vi "StartClone.vi"(7 "ShowPanel?":bool, 8 "error in (no error)":errorcluster, 10 "ModuleName":string="unnamed", 11 "VI Refnum":refnum<vi>) -> (0 "error out":errorcluster, 1 "FlagImpairBroadcast":T1, 3 "ModuleAdmin":refnum<class "ModuleAdmin.lvclass">)   [LabVIEW 2017, in "FlagImpairModule.lvlib"]
uses:
  FlagImpairModule.lvlib
  Protected/Broadcasts/clBroadcastEvents.ctl
  Protected/clEventType.ctl
  <userlib>/NIST/ModuleAdminLib/ModuleAdmin/ModuleAdmin.lvclass
  C:/Program Files (x86)/National Instruments/LabVIEW 2017/user.lib/NIST/ModuleAdminLib/ModuleAdminBase/ModuleAdminBase.lvclass
  <userlib>/NIST/ModuleAdminLib/CloneRegistration/CloneRegistration.lvclass
  <userlib>/NIST/ModuleAdminLib/ModuleAdmin/ModuleAdmin.lvclass/ModuleAdmin.ctl
  <userlib>/NIST/ModuleAdminLib/ModuleAdmin/Accessors/Write CloneRegRef.vi
  <userlib>/NIST/ModuleAdminLib/ModuleAdmin/Accessors/Write ShowPanel_.vi
  <vilib>/Utility/error.llb/Error Cluster From Error Code.vi
  <vilib>/ErrorRing/Error Ring.xnode
panel:
  # "If you want to add other Broadcast Events, open this typedef, copy an existing event and rename it to your event name.\n\nNext create an \"arg\" typedef for the  data and put it into PublicAPI/Arguments/Broadcasts\n\nAfter that, you will need to create a new roadcast vi in Protected/Broadcast.  Look at DidInit.vi or the reportError.vi as examples."
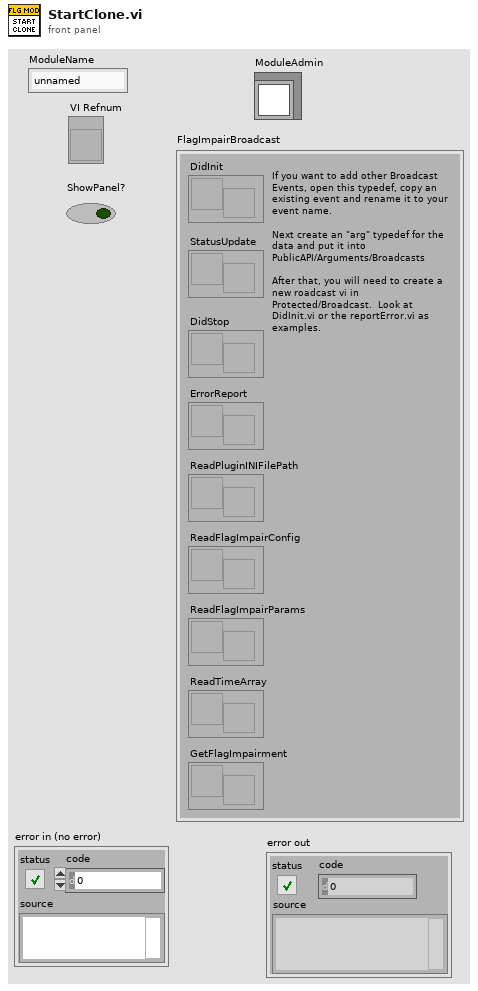
[diagram p1: front panel]
types:
  T1 = typedef "FlagImpairModule.lvlib/clBroadcastEvents.ctl" = cluster{"DidInit":refnum<user-event>, "StatusUpdate":refnum<user-event>, "ErrorReport":refnum<user-event>, "DidStop":refnum<user-event>, "ReadFlagImpairConfig":refnum<user-event>, "ReadPluginINIFilePath":refnum<user-event>, "ReadFlagImpairParams":refnum<user-event>, "ReadTimeArray":refnum<user-event>, "GetFlagImpairment":refnum<user-event>}
  T2 = enum32{"Bad", "Idle", "Run top level", "Running"}
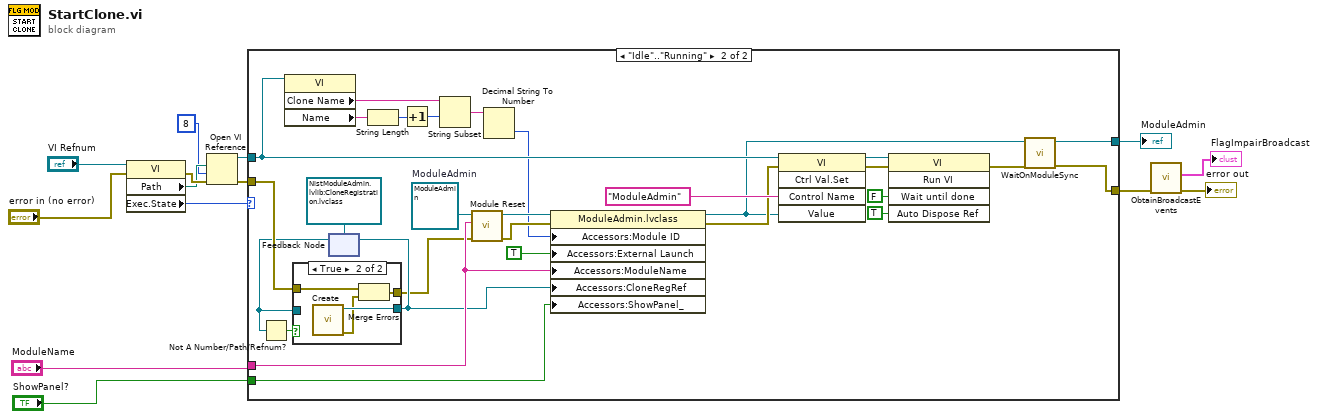
[diagram p0: block diagram]
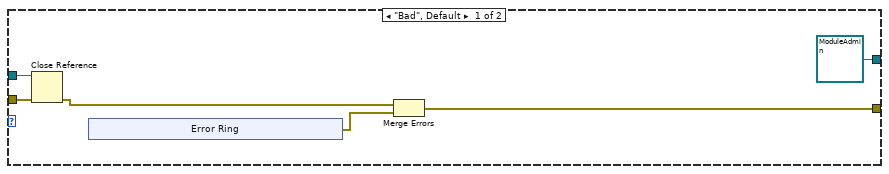
[diagram p2: hidden frame]
diagram:
  n1 = property class="VI"(reference="VI Refnum", error in="error in (no error)") -> (error out=w12:errorcluster, "Path"=w11:path, "Exec.State"=w13:T2)  [unwired: 1 out]
  n2 = Open VI Reference(vi path=w11, options=8, error in (no error)=w12) -> (vi reference=w9:refnum<vi>, error out=w10:errorcluster)  [unwired: 3 in]
  n3 = case shown="\"Idle\"..\"Running\"" w13 {
    tunnel: w10 -> [w20 w30]
    tunnel: w9 -> [w19 w44]
    tunnel: [w16 w32] -> w6
    tunnel: "ModuleName" -> [_ w35]
    tunnel: [refnum<class "ModuleAdmin.lvclass"> refnum ("ModuleAdmin") w34] -> w2
    tunnel: "ShowPanel?" -> [_ w25]
    frame "Bad", Default {
      n4 = Close Reference(reference=w19, error in (no error)=w20) -> (error out=w18:errorcluster)
      n5 = xnode "Error Ring"() -> ("error out"=w17:errorcluster)
      n6 = Merge Errors(w18, w17) -> (w16:errorcluster)
    }
    frame "Idle".."Running" {
      w48 = refnum<class "ModuleAdmin.lvclass"> refnum  # ModuleAdmin
      n7 = property class="VI"(reference=w44) -> ("Clone Name"=w50:string, "Name"=w53:string)  [unwired: 1 in, 2 out]
      n8 = feedback #1(refnum<data-value> refnum ("CloneRegRef")) -> (w28:refnum<data-value>)
      n9 = Not A Number/Path/Refnum?(number/path/refnum=w28) -> (NaN/Path/Refnum?=w29:bool)
      n10 = case shown="True" w29 {
        tunnel: [w55 w59] -> w27
        tunnel: w28 -> [w55 _]
        tunnel: w30 -> [w54 w57]
        tunnel: [w54 w56] -> w26
        frame False {
        }
        frame True {
          n11 = call <userlib>:"Create.vi"() -> ("error out"=w58:errorcluster, "CloneRegRef"=w59:refnum<data-value>)  [unwired: 10 in]
          n12 = Merge Errors(w57, w58) -> (w56:errorcluster)
        }
      }
      n13 = feedback-in #1(w27) -> ()
      n14 = String Length(string=w53) -> (length=w52:i32)
      n15 = Increment(x=w52) -> (x+1=w51:i32)
      n16 = String Subset(string=w50, offset (0)=w51) -> (substring=w49:string)  [unwired: 1 in]
      n17 = call <userlib>:"Module Reset.vi"("error in (no error)"=w26, "ModuleName"=w35, "Mod Admin in"=w48) -> ("error out"=w47:errorcluster, "Mod Admin out"=w46:refnum<class "ModuleAdmin.lvclass">)  [unwired: 7 in]
      n18 = Decimal String To Number(string=w49) -> (number=w36:i32)  [unwired: 2 in, 1 out]
      n19 = property class="ModuleAdmin.lvclass"(reference=w46, error in=w47, "Accessors:Module ID"=w36, "Accessors:External Launch"=TRUE ("External Launch"), "Accessors:ModuleName"=w35, "Accessors:CloneRegRef"=w27, "Accessors:ShowPanel_"=w25) -> (reference out=w33:refnum<class "ModuleAdmin.lvclass">, error out=w37:errorcluster)
      n20 = invoke class="VI" method="Ctrl Val.Set"(reference=w44, error in=w37, "Control Name"="ModuleAdmin", "Value"=w33) -> (reference out=w42:refnum<vi>, error out=w41:errorcluster)  [unwired: 1 in, 3 out]
      n21 = invoke class="VI" method="Run VI"(reference=w42, error in=w41, "Wait until done"=FALSE ("Wait Until Done"), "Auto Dispose Ref"=TRUE ("Auto Dispose Reference")) -> (error out=w38:errorcluster)  [unwired: 1 in, 4 out]
      n22 = call <userlib>:"WaitOnModuleSync.vi"("error in (no error)"=w38, "ModuleAdmin"=w33) -> ("error out"=w32:errorcluster, "ModuleAdmin"=w34:refnum<class "ModuleAdmin.lvclass">)  [unwired: 8 in]
    }
  }
  "ModuleAdmin" <- w2
  n23 = call "ObtainBroadcastEvents.vi"("error in (no error)"=w6) -> ("error out"=→"error out":errorcluster, "clBroadcastEvents"=→"FlagImpairBroadcast":T1)  [unwired: 9 in]
